vi "Read Hab Driver Operation.vi"(8 "Command Info":T3) -> (0 "Command Info":T3, 1 "SubSystem Data":T1, 2 "Command Timing":cluster{"Start Time (ms)":u32, "Iterations":i32})   [LabVIEW 2018]
doc: "This returns the most recently scheduled command. This doesn't indicate whether the command finished and is running the default command."
uses:
  <vilib>/Rock Robotics/WPI/Framework/Command Status Info.ctl
  <vilib>/Rock Robotics/WPI/Framework/Completion Status.ctl
  <vilib>/Rock Robotics/WPI/Framework/Completion Notifier.ctl
  Implementation/Hab Driver Setpoints.ctl
  Implementation/Hab Driver Operations.ctl
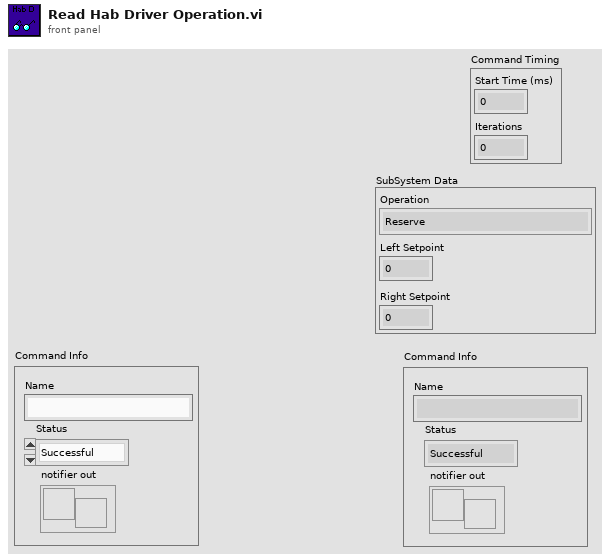
[diagram p1: front panel]
types:
  T1 = typedef "Hab Driver Setpoints.ctl" = cluster{"Operation":T2, "Left Setpoint":dbl, "Right Setpoint":dbl}
  T2 = typedef "Hab Driver Operations.ctl" = enum16{"Reserve", "Read Current", "Immediate", "Emma: Drive around with the extendo wheels"}
  T3 = typedef "Command Status Info.ctl" = cluster{"Name":string, "Status":T4, "notifier out":T5}
  T4 = typedef "Completion Status.ctl" = enum16{"Successful", "Aborted", "Incomplete"}
  T5 = typedef "Completion Notifier.ctl" = refnum<notifier>
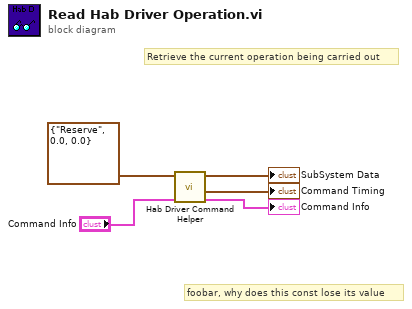
[diagram p0: block diagram]
diagram:
  # "foobar, why does this const lose its value"
  # "Retrieve the current operation being carried out"
  n1 = call "Hab Driver Command Helper.vi"("Command Info In"="Command Info", "SubSystem Data"=T1 {"Operation"=enum."Reserve", "Left Setpoint"=0.0, "Right Setpoint"=0.0}) -> ("Command Info Out"=→"Command Info":T3, "Command Timing"=→"Command Timing":cluster{"Start Time (ms)":u32, "Iterations":i32}, "SubSystem Data"=→"SubSystem Data":T1)  [unwired: 7 in]
